vi "Save As.vi"(8 "error in (no error)":errorcluster, 11 "Config Name":string) -> (0 "error out":errorcluster)   [LabVIEW 2015, in "System Config.lvclass"]
uses:
  System Config.lvclass
  <vilib>/Utility/config.llb/NI_LVConfig.lvlib
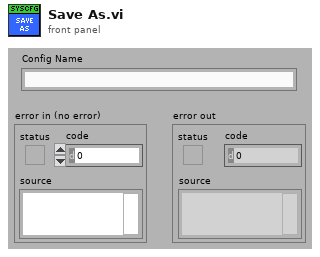
[diagram p1: front panel]
types:
  T1 = typedef "System Config.lvclass/ClassAttributesRef.ctl" = refnum<data-value>
  T2 = typedef "System Config.lvclass/ClassAttributes.ctl" = cluster{"Config":cluster{"Logging":cluster{"Log Files Directory":path, "Max Lines Per Log File":i32}, "Settings":T3}, "Core":cluster{"Config Directory":path, "Name":string, "Config Changed":refnum<user-event>}}
  T3 = typedef "System Config.lvclass/Settings.ctl" = cluster{"Dummy":dbl}
  T4 = cluster{"Logging":cluster{"Log Files Directory":path, "Max Lines Per Log File":i32}, "Settings":T3}
  T5 = typedef "NI_LVConfig.lvlib/Config Data RefNum.ctl" = refnum<k1>
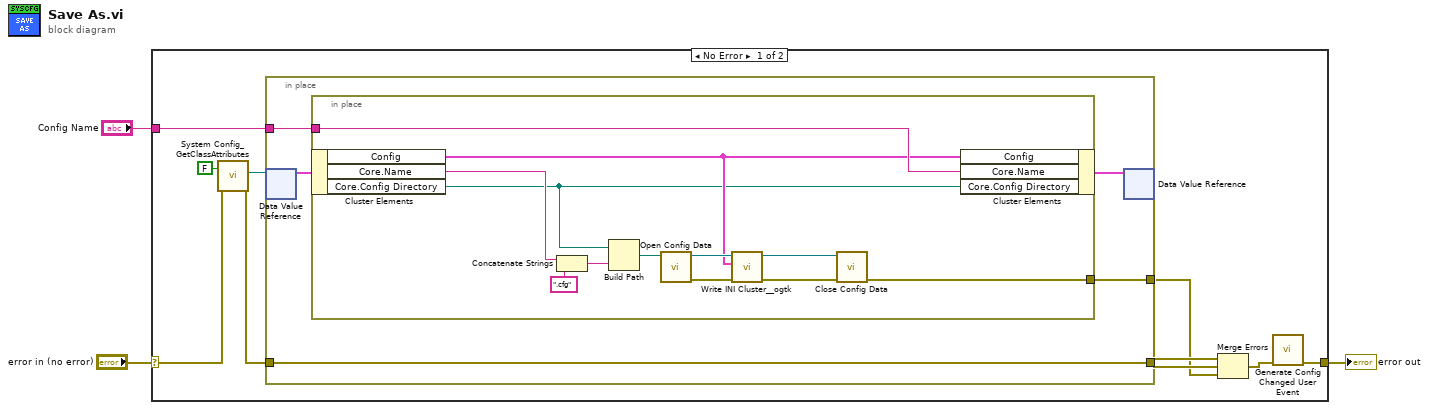
[diagram p0: block diagram]
diagram:
  n1 = case shown="No Error" "error in (no error)" {
    selector: "error in (no error)" -> [w13 w31]
    tunnel: [w5 w31] -> w2
    tunnel: "Config Name" -> [w7 _]
    frame No Error {
      n2 = call "System Config_GetClassAttributes.vi"("error in (no error)"=w13, "return data? (T)"=FALSE ("return data")) -> ("error out"=w12:errorcluster, "class attributes ref"=w11:T1)  [unwired: 6 in, 2 out]
      n3 = in-place {
        in-place-border: w12 -> [w16]
        in-place-border: [w16] -> w9
        in-place-border: w7 -> [w15]
        in-place-border: [w14] -> w4
        n4 = in-place-dvr #1(w11) -> (w17:T2)  [unwired: 1 out]
        n5 = in-place {
          in-place-border: w15 -> [w30]
          in-place-border: [w21] -> w14
          n6 = in-place-cluster #2(w17) -> ("Config"=w20:T4, "Core.Name"=w29:string, "Core.Config Directory"=w19:path)
          n7 = Concatenate Strings(w29, ".cfg" ("string")) -> (w27:string)
          n8 = Build Path(base path=w19, name or relative path=w27) -> (appended path=w26:path)
          n9 = call <vilib>:"Open Config Data.vi"("configuration file path"=w26) -> ("error out"=w23:errorcluster, "refnum"=w25:T5)  [unwired: 8 in, 1 out]
          n10 = call <userlib>:"Write INI Cluster__ogtk.vi"("error in (no error)"=w23, "INI Fomatted Cluster"=w20, "refnum"=w25) -> ("error out"=w22:errorcluster, "dup refnum"=w24:T5)  [unwired: 7 in]
          n11 = call <vilib>:"Close Config Data.vi"("error in (no error)"=w22, "refnum"=w24) -> ("error out"=w21:errorcluster)  [unwired: 8 in, 1 out]
          n12 = in-place-cluster #2("Config"=w20, "Core.Name"=w30, "Core.Config Directory"=w19) -> (w18:T2)
        }
        n13 = in-place-dvr #1(w18) -> (w8:errorcluster)  [unwired: 1 out]
      }
      n14 = Merge Errors(w9, w8, w4) -> (w6:errorcluster)
      n15 = call "Generate Config Changed User Event.vi"("error in (no error)"=w6) -> ("error out"=w5:errorcluster)  [unwired: 10 in]
    }
    frame Error {
    }
  }
  "error out" <- w2
